vi "Escape HTTP URL String.vi"(1 "Unescaped HTTP URL string in":string) -> (0 "Escaped HTTP URL string out":string)   [LabVIEW 2018, in "REST Client_JKI.lvlib" / "REST Client.lvclass"]
doc: "Escape URL string."
uses:
  REST Client.lvclass
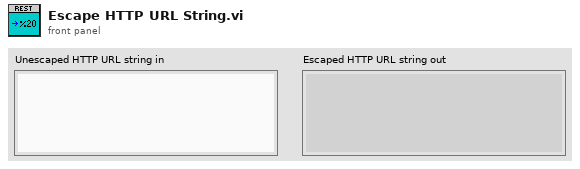
[diagram p1: front panel]
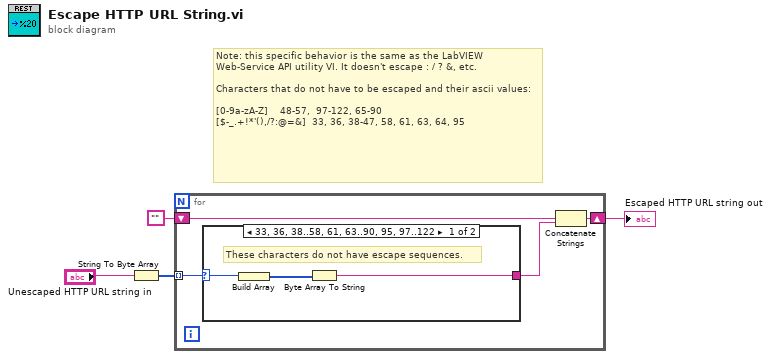
[diagram p0: block diagram]
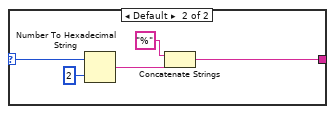
[diagram p2: hidden frame]
diagram:
  # "Note: this specific behavior is the same as the LabVIEW Web-Service API utility VI. It doesn't escape : / ? &, etc.\n\nCharacters that do not have to be escaped and their ascii values:\n\n[0-9a-zA-Z]    48-57,  97-122, 65-90 \n[$-_.+!*'(),/?:@=&]  33, 36, 38-47, 58, 61, 63, 64, 95"
  n1 = String To Byte Array(string="Unescaped HTTP URL string in") -> (unsigned byte array=w1:u8[])
  n2 = for {
    shift-right: [w5] -> w4
    shift-left: "" -> [w6]
    tunnel: w1 -> [w8] mode=indexing
    n3 = case shown="33, 36, 38..58, 61, 63..90, 95, 97..122" w8 {
      selector: w8 -> [w11 w14]
      tunnel: [w9 w13] -> w7
      frame 33, 36, 38..58, 61, 63..90, 95, 97..122 {
        # "These characters do not have escape sequences."
        n4 = Build Array(w11) -> (w10:u8[])
        n5 = Byte Array To String(unsigned byte array=w10) -> (string=w9:string)
      }
      frame Default {
        n6 = Number To Hexadecimal String(1:i16 2 ("width (-)"), 2:w14) -> (0:w15:string)
        n7 = Concatenate Strings("%" ("string"), w15) -> (w13:string)
      }
    }
    n8 = Concatenate Strings(w6, w7) -> (w5:string)
  }
  "Escaped HTTP URL string out" <- w4
